vi "reflectivity_to_pixmap_TOF_.vi"(5 "Custom Colours":u32[](array[colorbox]), 6 "colours":T1(ring), 8 "min value":dbl=nan, 9 "max value":dbl=nan, 10 "DBL Array":dbl[][](array[numeric])) -> (3 "image data":T2)   [LabVIEW 2020]
uses:
  <vilib>/picture/picture.llb/imagedata.ctl
panel:
  out "output array":u32[](array[numeric])
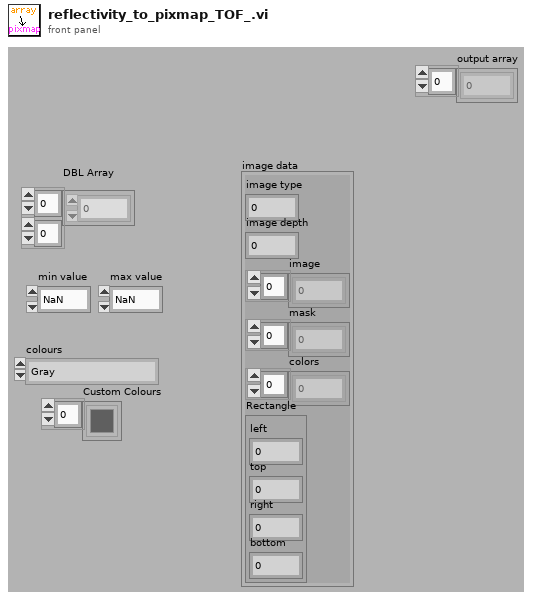
[diagram p1: front panel]
types:
  T1 = enum16{"Gray", "RGB", "CMY", "Black -> Blue -> White", "Custom", "HSL"}
  T2 = typedef "imagedata.ctl" = cluster{"image type":i32, "image depth":i32, "image":u8[], "mask":u8[], "colors":u32[], "Rectangle":cluster{"left":i16, "top":i16, "right":i16, "bottom":i16}}
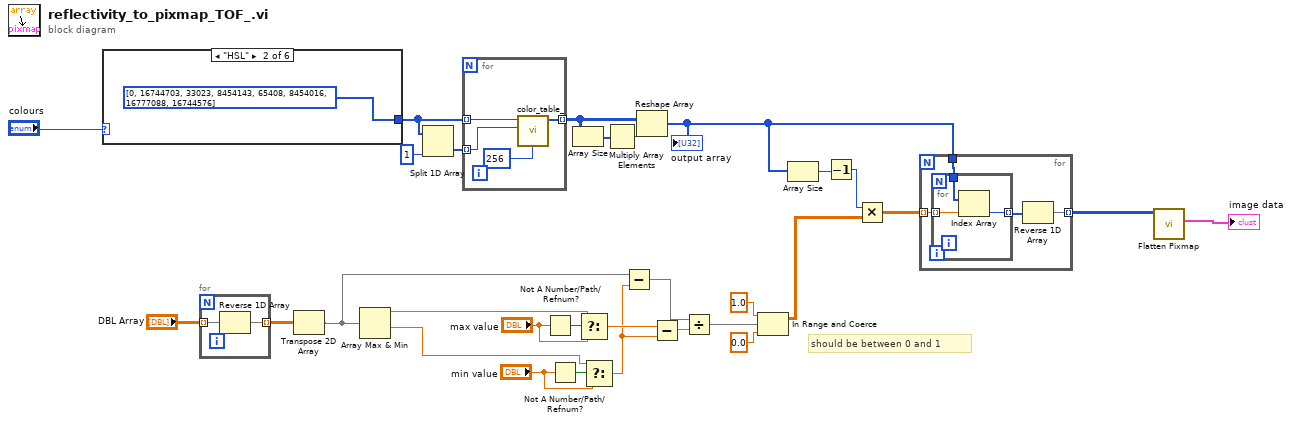
[diagram p0: block diagram]
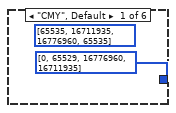
[diagram p2: hidden frame]
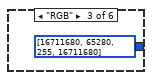
[diagram p3: hidden frame]
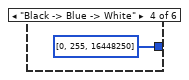
[diagram p4: hidden frame]
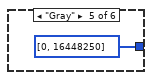
[diagram p5: hidden frame]
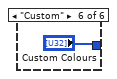
[diagram p6: hidden frame]
diagram:
  # "should be between 0 and 1"
  n1 = case shown="\"HSL\"" "colours" {
    tunnel: [u32[] [0, 65529, 16776960, 16711935] u32[] [0, 16744703, 33023, 8454143, 65408, 8454016, 16777088, 16744576] u32[] [16711680, 65280, 255, 16711680] u32[] [0, 255, 16448250] u32[] [0, 16448250] "Custom Colours"] -> w24
    frame "CMY", Default {
      (unwired) u32[] [65535, 16711935, 16776960, 65535]
    }
    frame "HSL" {
    }
    frame "RGB" {
    }
    frame "Black -> Blue -> White" {
    }
    frame "Gray" {
    }
    frame "Custom" {
    }
  }
  n2 = for {
    tunnel: "DBL Array" -> [w38] mode=indexing
    tunnel: [w37] -> w6 mode=indexing
    n3 = Reverse 1D Array(array=w38) -> (reversed array=w37:dbl[])
  }
  n4 = Transpose 2D Array(2D array=w6) -> (transposed array=w2:dbl[][])
  n5 = Array Max & Min(array=w2) -> (max value=w18:dbl, min value=w15:dbl)  [unwired: 2 out]
  n6 = Split 1D Array(array=w24, index=1) -> (second subarray=w25:u32[])  [unwired: 1 out]
  n7 = for {
    tunnel: w25 -> [w40] mode=indexing
    tunnel: w24 -> [w41] mode=indexing
    tunnel: [w39] -> w23 mode=indexing
    n8 = call "color_table_.vi"("N"=256, "Color 2"=w40, "Color 1"=w41) -> ("Color Table (element 0=color 1, element N-1=color 2)"=w39:u32[])  [unwired: 8 in]
  }
  n9 = Not A Number/Path/Refnum?(number/path/refnum="max value") -> (NaN/Path/Refnum?=w19:bool)
  n10 = Not A Number/Path/Refnum?(number/path/refnum="min value") -> (NaN/Path/Refnum?=w16:bool)
  n11 = Array Size(array=w23) -> (size(s)=w22:i32[])
  n12 = Select(t=w18, s=w19, f="max value") -> (s? t:f=w13:dbl)
  n13 = Select(t=w15, s=w16, f="min value") -> (s? t:f=w10:dbl)
  n14 = Multiply Array Elements(1:w22) -> (0:w21:i32)
  n15 = Subtract(x=w2, y=w10) -> (x-y=w3:dbl[][])
  n16 = Reshape Array(w23, w21) -> (w20:u32[])
  "output array" <- w20
  n17 = Subtract(x=w13, y=w10) -> (x-y=w12:dbl)
  n18 = Divide(x=w3, y=w12) -> (x/y=w4:dbl[][])
  n19 = In Range and Coerce(upper limit=1.0 ("max value"), x=w4, lower limit=0.0 ("max value")) -> (coerced(x)=w1:dbl[][])  [unwired: 1 out]
  n20 = Array Size(array=w20) -> (size(s)=w27:i32)
  n21 = Decrement(x=w27) -> (x-1=w11:i32)
  n22 = Multiply(x=w11, y=w1) -> (x*y=w9:dbl[][])
  n23 = for {
    tunnel: [w45] -> w29 mode=indexing
    tunnel: w20 -> [w44]
    tunnel: w9 -> [w43] mode=indexing
    n24 = for {
      tunnel: [w49] -> w46 mode=indexing
      tunnel: w44 -> [w48]
      tunnel: w43 -> [w47] mode=indexing
      n25 = Index Array(array=w48, index=w47) -> (element=w49:u32)
    }
    n26 = Reverse 1D Array(array=w46) -> (reversed array=w45:u32[])
  }
  n27 = call <vilib>:"Flatten Pixmap.vi"("24-bit pixmap"=w29) -> ("image data"=→"image data":T2)  [unwired: 10 in]
